vi "Reasons For Termination Data Decode.vi"(7 "Data":u16(ring) items=["Data1", "Data2", "Data3", "Data4"], 10 "Reason for Last Heating Cycle Termination":u16, 11 "Reason Data Word":string) -> (3 "Reason Data Word 1 Output":string)   [LabVIEW 2016]
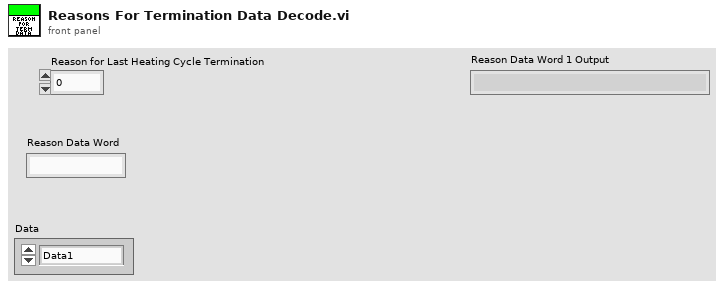
[diagram p1: front panel]
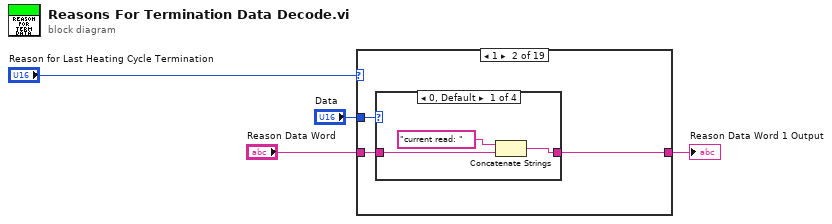
[diagram p0: block diagram]
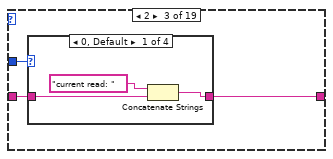
[diagram p6: hidden frame]
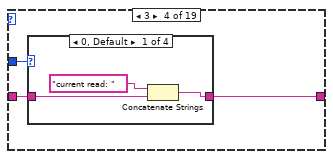
[diagram p10: hidden frame]
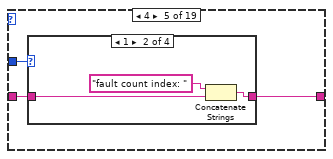
[diagram p14: hidden frame]
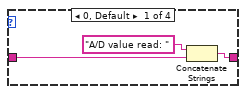
[diagram p15: hidden frame]
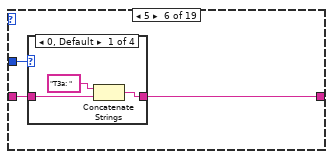
[diagram p18: hidden frame]
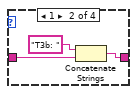
[diagram p19: hidden frame]
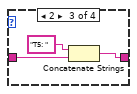
[diagram p20: hidden frame]
diagram:
  n1 = case shown="1" "Reason for Last Heating Cycle Termination" {
    tunnel: "Reason Data Word" -> [w5 w8 w17 w25 w35 w45 w58 w72 w81 w90 w104 w120 w131 w142 w151 w164 w173 w184 w193]
    tunnel: [w5 w7 w16 w26 w34 w44 w57 w71 w80 w89 w105 w119 w130 w141 w150 w163 w172 w183 w192] -> w2
    tunnel: "Data" -> [_ w6 w15 w24 w33 w46 w59 w70 w79 w88 w103 w118 w129 w140 w149 w162 w171 w182 w191]
    frame 0, Default {
    }
    frame 1 {
      n2 = case shown="0, Default" w6 {
        tunnel: w8 -> [w10 w12 w13 w14]
        tunnel: [w9 w12 w13 w14] -> w7
        frame 0, Default {
          n3 = Concatenate Strings("current read: " ("string"), w10) -> (w9:string)
        }
        frame 1 {
        }
        frame 2 {
        }
        frame 3 {
        }
      }
    }
    frame 2 {
      n4 = case shown="0, Default" w15 {
        tunnel: w17 -> [w19 w21 w22 w23]
        tunnel: [w18 w21 w22 w23] -> w16
        frame 0, Default {
          n5 = Concatenate Strings("current read: " ("string"), w19) -> (w18:string)
        }
        frame 1 {
        }
        frame 2 {
        }
        frame 3 {
        }
      }
    }
    frame 3 {
      n6 = case shown="0, Default" w24 {
        tunnel: w25 -> [w28 w30 w31 w32]
        tunnel: [w27 w30 w31 w32] -> w26
        frame 0, Default {
          n7 = Concatenate Strings("current read: " ("string"), w28) -> (w27:string)
        }
        frame 1 {
        }
        frame 2 {
        }
        frame 3 {
        }
      }
    }
    frame 4 {
      n8 = case shown="1" w33 {
        tunnel: w35 -> [w37 w39 w42 w43]
        tunnel: [w36 w41 w42 w43] -> w34
        frame 0, Default {
          n9 = Concatenate Strings("A/D value read: " ("string"), w37) -> (w36:string)
        }
        frame 1 {
          n10 = Concatenate Strings("fault count index: " ("string"), w39) -> (w41:string)
        }
        frame 2 {
        }
        frame 3 {
        }
      }
    }
    frame 5 {
      n11 = case shown="0, Default" w46 {
        tunnel: w45 -> [w48 w51 w54 w56]
        tunnel: [w47 w50 w53 w56] -> w44
        frame 0, Default {
          n12 = Concatenate Strings("T3a: " ("string"), w48) -> (w47:string)
        }
        frame 1 {
          n13 = Concatenate Strings("T3b: " ("string"), w51) -> (w50:string)
        }
        frame 2 {
          n14 = Concatenate Strings("T5: " ("string"), w54) -> (w53:string)
        }
        frame 3 {
        }
      }
    }
    frame 6 {
      n15 = case shown="3" w59 {
        tunnel: w58 -> [w61 w65 w68 w69]
        tunnel: [w60 w64 w67 w69] -> w57
        frame 0, Default {
          n16 = Concatenate Strings("T3a: " ("string"), w61) -> (w60:string)
        }
        frame 1 {
          n17 = Concatenate Strings("T2: " ("string"), w65) -> (w64:string)
        }
        frame 2 {
          n18 = Concatenate Strings("T5: " ("string"), w68) -> (w67:string)
        }
        frame 3 {
        }
      }
    }
    frame 7 {
      n19 = case shown="0, Default" w70 {
        tunnel: w72 -> [w74 w76 w77 w78]
        tunnel: [w73 w76 w77 w78] -> w71
        frame 0, Default {
          n20 = Concatenate Strings("Voltage read:" ("string"), w74) -> (w73:string)
        }
        frame 1 {
        }
        frame 2 {
        }
        frame 3 {
        }
      }
    }
    frame 8 {
      n21 = case shown="0, Default" w79 {
        tunnel: w81 -> [w83 w85 w86 w87]
        tunnel: [w82 w85 w86 w87] -> w80
        frame 0, Default {
          n22 = Concatenate Strings("Voltage read:" ("string"), w83) -> (w82:string)
        }
        frame 1 {
        }
        frame 2 {
        }
        frame 3 {
        }
      }
    }
    frame 9 {
      n23 = case shown="2" w88 {
        tunnel: w90 -> [w92 w96 w99 w101]
        tunnel: [w91 w95 w98 w100] -> w89
        frame 0, Default {
          n24 = Concatenate Strings("Resolved Set Point: " ("string"), w92) -> (w91:string)
        }
        frame 1 {
          n25 = Concatenate Strings("T2: " ("string"), w96) -> (w95:string)
        }
        frame 2 {
          n26 = Concatenate Strings("Turn on temp error: " ("string"), w99) -> (w98:string)
        }
        frame 3 {
          n27 = Concatenate Strings("Turn off temp error: " ("string"), w101) -> (w100:string)
        }
      }
    }
    frame 10 {
      n28 = case shown="2" w103 {
        tunnel: w104 -> [w107 w111 w114 w116]
        tunnel: [w106 w110 w113 w115] -> w105
        frame 0, Default {
          n29 = Concatenate Strings("Resolved Set Point: " ("string"), w107) -> (w106:string)
        }
        frame 1 {
          n30 = Concatenate Strings("T2: " ("string"), w111) -> (w110:string)
        }
        frame 2 {
          n31 = Concatenate Strings("Turn on temp error: " ("string"), w114) -> (w113:string)
        }
        frame 3 {
          n32 = Concatenate Strings("Turn off temp error: " ("string"), w116) -> (w115:string)
        }
      }
    }
    frame 11 {
      n33 = case shown="1" w118 {
        tunnel: w120 -> [w122 w126 w127 w128]
        tunnel: [w121 w125 w127 w128] -> w119
        frame 0, Default {
          n34 = Concatenate Strings("T4: " ("string"), w122) -> (w121:string)
        }
        frame 1 {
          n35 = Concatenate Strings("Initial T4: " ("string"), w126) -> (w125:string)
        }
        frame 2 {
        }
        frame 3 {
        }
      }
    }
    frame 12 {
      n36 = case shown="2" w129 {
        tunnel: w131 -> [w133 w137 w138 w139]
        tunnel: [w132 w136 w138 w139] -> w130
        frame 0, Default {
          n37 = Concatenate Strings("T4 (deg F tenths): " ("string"), w133) -> (w132:string)
        }
        frame 1 {
          n38 = Concatenate Strings("T5 (deg F): " ("string"), w137) -> (w136:string)
        }
        frame 2 {
        }
        frame 3 {
        }
      }
    }
    frame 13 {
      n39 = case shown="0, Default" w140 {
        tunnel: w142 -> [w144 w146 w147 w148]
        tunnel: [w143 w146 w147 w148] -> w141
        frame 0, Default {
          n40 = Concatenate Strings("T3a 15 minute average: " ("string"), w144) -> (w143:string)
        }
        frame 1 {
        }
        frame 2 {
        }
        frame 3 {
        }
      }
    }
    frame 14 {
      n41 = case shown="3" w149 {
        tunnel: w151 -> [w153 w157 w160 w161]
        tunnel: [w152 w155 w159 w161] -> w150
        frame 0, Default {
          n42 = Concatenate Strings("T3A: " ("string"), w153) -> (w152:string)
        }
        frame 1 {
          n43 = Concatenate Strings("T3b: " ("string"), w157) -> (w155:string)
        }
        frame 2 {
          n44 = Concatenate Strings("T5: " ("string"), w160) -> (w159:string)
        }
        frame 3 {
        }
      }
    }
    frame 15 {
      n45 = case shown="1" w162 {
        tunnel: w164 -> [w166 w168 w169 w170]
        tunnel: [w165 w168 w169 w170] -> w163
        frame 0, Default {
          n46 = Concatenate Strings("T4: " ("string"), w166) -> (w165:string)
        }
        frame 1 {
        }
        frame 2 {
        }
        frame 3 {
        }
      }
    }
    frame 16 {
      n47 = case shown="1" w171 {
        tunnel: w173 -> [w175 w179 w180 w181]
        tunnel: [w174 w178 w180 w181] -> w172
        frame 0, Default {
          n48 = Concatenate Strings("EEV position when faulted: " ("string"), w175) -> (w174:string)
        }
        frame 1 {
          n49 = Concatenate Strings("PID change in position: " ("string"), w179) -> (w178:string)
        }
        frame 2 {
        }
        frame 3 {
        }
      }
    }
    frame 17 {
      n50 = case shown="1" w182 {
        tunnel: w184 -> [w186 w188 w189 w190]
        tunnel: [w185 w188 w189 w190] -> w183
        frame 0, Default {
          n51 = Concatenate Strings("T5: " ("string"), w186) -> (w185:string)
        }
        frame 1 {
        }
        frame 2 {
        }
        frame 3 {
        }
      }
    }
    frame 18 {
      n52 = case shown="3" w191 {
        tunnel: w193 -> [w195 w199 w202 w203]
        tunnel: [w194 w198 w201 w203] -> w192
        frame 0, Default {
          n53 = Concatenate Strings("T5: " ("string"), w195) -> (w194:string)
        }
        frame 1 {
          n54 = Concatenate Strings("Voltage: " ("string"), w199) -> (w198:string)
        }
        frame 2 {
          n55 = Concatenate Strings("Current (amps x 10): " ("string"), w202) -> (w201:string)
        }
        frame 3 {
        }
      }
    }
  }
  "Reason Data Word 1 Output" <- w2
